vi "Generate daily results folder name.vi"() -> (1 "Generated daily folder name":string="2015-May-21")   [LabVIEW 2017]
panel:
  in  "Date format (short)":enum16{"short", "long", "abbreviated"}(ring)
  in  "Year first (T)":bool=TRUE
  in  "Want seconds? (T)":bool=TRUE
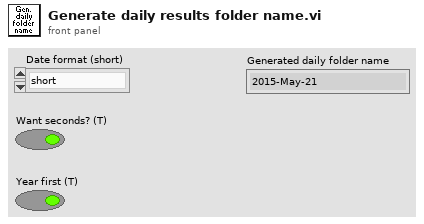
[diagram p1: front panel]
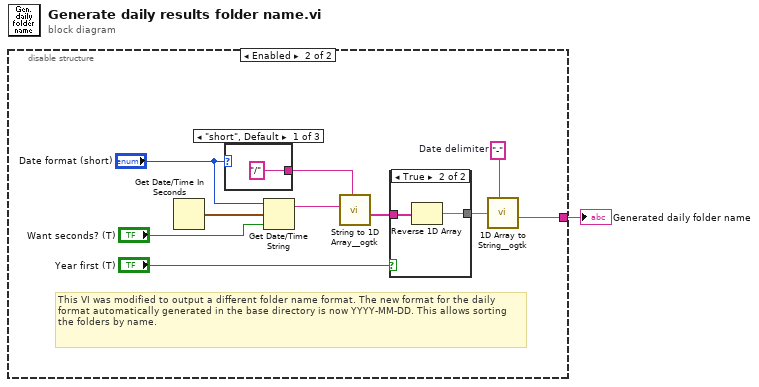
[diagram p0: block diagram]
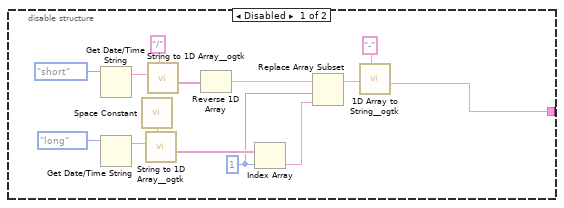
[diagram p2: hidden frame]
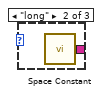
[diagram p4: hidden frame]
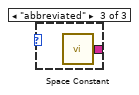
[diagram p5: hidden frame]
diagram:
  n1 = disable-structure shown="Enabled" {
    disable-tunnel: [w2 w16] -> w1
    frame Disabled {
      w3 = 1 ("index")
      n2 = Get Date/Time String(date format (0)=enum16{"short", "long", "abbreviated"}."short") -> (date string=w14:string)  [unwired: 2 in, 1 out]
      n3 = Get Date/Time String(date format (0)=enum16{"short", "long", "abbreviated"}."long") -> (date string=w8:string)  [unwired: 2 in, 1 out]
      n4 = call <vilib>:"Space Constant.vi"() -> ("String"=w9:string)
      n5 = call <userlib>:"String to 1D Array__ogtk.vi"("delimiter (Tab)"=w9, "string"=w8) -> ("Array of Strings"=w7:string[])  [unwired: 9 in]
      n6 = call <userlib>:"String to 1D Array__ogtk.vi"("delimiter (Tab)"="/", "string"=w14) -> ("Array of Strings"=w12:string[])  [unwired: 9 in]
      n7 = Reverse 1D Array(array=w12) -> (reversed array=w6:string[])
      n8 = Index Array(array=w7, index=w3) -> (element=w4:string)
      n9 = Replace Array Subset(array=w6, new element=w4, index=w3) -> (w5:string[])
      n10 = call <userlib>:"1D Array to String__ogtk.vi"("delimiter (Tab)"="-", "Array of Strings"=w5) -> ("delimited string"=w2:string)  [unwired: 9 in]
    }
    frame Enabled {
      w22 = "-"  # Date delimiter
      # "This VI was modified to output a different folder name format. The new format for the daily format automatically generated in the base directory is now YYYY-MM-DD. This allows sorting the folders by name."
      n11 = Get Date/Time In Seconds() -> (seconds since 1Jan1904=w18:timestamp)
      n12 = case shown="\"short\", Default" "Date format (short)" {
        tunnel: ["/" ("delimiter (Tab)") w30 w31] -> w24
        frame "short", Default {
        }
        frame "long" {
          n13 = call <vilib>:"Space Constant.vi"() -> ("String"=w30:string)
        }
        frame "abbreviated" {
          n14 = call <vilib>:"Space Constant.vi"() -> ("String"=w31:string)
        }
      }
      n15 = Get Date/Time String(date format (0)="Date format (short)", seconds (now)=w18, want seconds? (F)="Want seconds? (T)") -> (date string=w19:string)  [unwired: 1 out]
      n16 = call <userlib>:"String to 1D Array__ogtk.vi"("delimiter (Tab)"=w24, "string"=w19) -> ("Array of Strings"=w20:string[])  [unwired: 9 in]
      n17 = case shown="True" "Year first (T)" {
        tunnel: [w26 w28] -> w21
        tunnel: w20 -> [w26 w27]
        frame False {
        }
        frame True {
          n18 = Reverse 1D Array(array=w27) -> (reversed array=w28:string[])
        }
      }
      n19 = call <userlib>:"1D Array to String__ogtk.vi"("delimiter (Tab)"=w22, "Array of Strings"=w21) -> ("delimited string"=w16:string)  [unwired: 9 in]
    }
  }
  "Generated daily folder name" <- w1
